vi "Control Loop.vi"(10 "Queue":refnum<queue>) -> ()   [LabVIEW 2021]
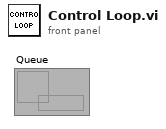
[diagram p1: front panel]
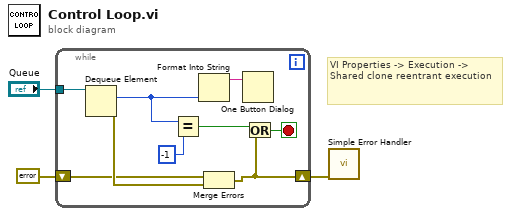
[diagram p0: block diagram]
diagram:
  # "VI Properties -> Execution -> Shared clone reentrant execution"
  n1 = while {
    tunnel: "Queue" -> [w7]
    shift-right: [w4] -> w2
    shift-left: errorcluster {"status"=FALSE, "code"=0, "source"=""} ("error IO") -> [w6]
    stop <- w5 stop-if-true
    n2 = Dequeue Element(queue=w7) -> (element=w8:i32, error out=w10:errorcluster)  [unwired: 2 in, 2 out]
    n3 = Equal?(x=w8, y=-1) -> (x = y?=w12:bool)
    n4 = Format Into String(w8) -> (resulting string=w9:string)  [unwired: 3 in, 1 out]
    n5 = Merge Errors(w6, w10) -> (w4:errorcluster)
    n6 = One Button Dialog(message=w9) -> ()  [unwired: 1 in, 1 out]
    n7 = Or(x=w12, y=w4) -> (x .or. y?=w5:bool)
  }
  n8 = call <vilib>:"Simple Error Handler.vi"("error in (no error)"=w2) -> ()  [unwired: 4 in, 5 out]
